vi "Config Type.vi"(11 "Reset Var Command in":refnum<class "Reset Var Command.lvclass">) -> (2 "Command Config Type":refnum<class "Command Config.lvclass">)   [LabVIEW 2020, in "VolatusSeq.lvlib" / "Reset Var Command.lvclass"]
uses:
  Reset Var Command.lvclass
  Reset Var Command.lvclass/Reset Var Command.ctl
  VolatusSeqConfig/Reset Var Command Config/Reset Var Command Config.lvclass
  C:/dev/lv20CE/relink/lv-volatus/VolatusSeqConfig/Command Config/Command Config.lvclass
  C:/dev/lv20CE/relink/lv-volatus/VolatusSeqConfig/Reset Var Command Config/Reset Var Command Config.lvclass
  VolatusSeqConfig/Command Config/Command Config.lvclass
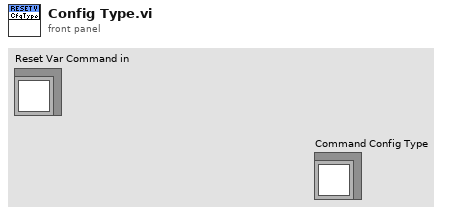
[diagram p1: front panel]
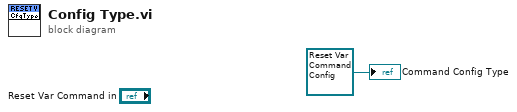
[diagram p0: block diagram]
diagram:
  "Command Config Type" <- refnum<class "Reset Var Command Config.lvclass"> refnum ("VolatusSeqConfig.lvlib:Reset Var Command Config.lvclass")
